vi "Display.vi"(10 "EnableDisplay":bool, 11 "Photometrics Cam v2 in":refnum<class "Photometrics_CH-250_Cam.lvclass">) -> (2 "TReading(DegC)":dbl, 3 "PropertyDefinition:New Image":T1)   [LabVIEW 2013, in "Photometrics_CH-250_Cam.lvclass"]
uses:
  Photometrics_CH-250_Cam.lvclass
  <vilib>/vision/Image Controls.llb/IMAQ Image.ctl
  Photometrics_CH-250_Cam.lvclass/Photometrics_CH-250_Cam.ctl
  CameraSessionClass/CS250-CameraHardwareClass.lvclass
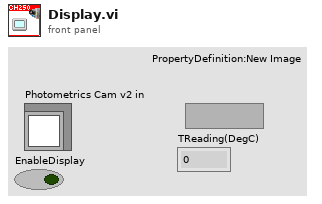
[diagram p1: front panel]
types:
  T1 = typedef "IMAQ Image.ctl" = refnum<image>
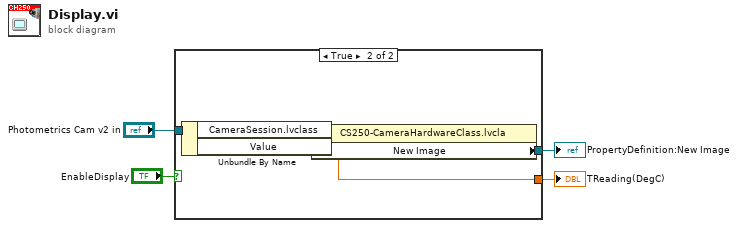
[diagram p0: block diagram]
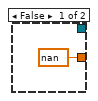
[diagram p2: hidden frame]
diagram:
  n1 = case shown="True" "EnableDisplay" {
    tunnel: [_ w9] -> w4
    tunnel: "Photometrics Cam v2 in" -> [_ w7]
    tunnel: [nan ("Value") w6] -> w1
    frame False {
    }
    frame True {
      n2 = Unbundle By Name(w7) -> ("CameraSession.lvclass"=w8:refnum<class "CS250-CameraHardwareClass.lvclass">, "Value"=w6:dbl)
      n3 = property class="CS250-CameraHardwareClass.lvcla"(reference=w8) -> ("New Image"=w9:T1)  [unwired: 1 in, 2 out]
    }
  }
  "PropertyDefinition:New Image" <- w4
  "TReading(DegC)" <- w1
